vi "Lab6_template_v1.0.vi"() -> ()   [LabVIEW 2018]
doc: "Main VI for the controls"
uses:
  components/PMCL Dynamic Signal Analyzer/Controls/DSA excitation specs.ctl
  components/PMCL Dynamic Signal Analyzer/Controls/DSA cycle specs.ctl
  Typedefs/StateDef_Enum.ctl
  <vilib>/Utility/error.llb/DialogType.ctl
  components/Motor Read Angle/Task cluster.ctl
  <vilib>/Platform/TimedLoop/XDataNode/timing_clust.ctl
  <vilib>/Platform/TimedLoop/XDataNode/nitl_modes.ctl
  <vilib>/Platform/TimedLoop/XDataNode/wakeup.ctl
  <vilib>/DAQmx/write.llb/DAQmx Write (Analog 1D DBL NChan 1Samp).vi
  <vilib>/DAQmx/create/channels.llb/DAQmx Create Channel (AO-Voltage-Basic).vi
  <vilib>/DAQmx/miscellaneous.llb/DAQmx Fill In Error Info.vi
  <vilib>/platform/TimedLoop/XDataNode/XDataNode.xnode
  Components/Timing/Timing.lvlib
  <vilib>/Platform/TimedLoop/XDataNode/XDNodeRunTimeDep.lvlib
  <vilib>/Analysis/NI_AALPro.lvlib
  <vilib>/ptbypt/NI_PtbyPt.lvlib
  Components/Controller/Controller.lvlib
  components/Motor Read Angle/Motor_ReadAng.lvlib
panel:
  in  "System Stop Button":bool
  in  "Pause chart?":bool
  in  "Controller Params":enum32{"Page 1"}(tab)
  in  "Kp":dbl=1.0 min=0.0
  in  "Controller On?":bool
  out "Found index?":bool
  out "Status":string="Stopped."
  in  "Ref. Gen.":T1(tab)=enum."Manual"
  in  "Ref. cmd.":dbl(slide) caption="Ref. cmd. [deg.]" step=1.0 scale=-90.0..90.0 scale format="%#.1f"
  in  "Signal Cluster":T2={"phase"=0.0, "amplitude"=1.0, "frequency"=1.0, "offset"=1.0, "Signal"=enum."Square"} {"offset" format="%0.2f"; "frequency" format="%0.2f"; "amplitude" format="%0.2f"; "phase" format="%0.2f"}
  in  "Frequency\nResponse":enum16{"Plant", "RR", "CL"}(ring)
  out "DSA \nRunning?":bool
  in  "Stop \nDSA":bool
  in  "Start \nDSA":bool
  in  "DSA excitation specs":T3={"Initial Freq. [Hz]"=10.0, "Final Freq. [Hz]"=999.0, "# pts. in interval"=50, "Samping Time [s]"=0.000333, "Amplitude [V]"=1.0, "Offset [V]"=0.0, "Freq Units (F: rad/s, T: Hz)"=TRUE}
  in  "Cycle Specs":T4={"Cycles To \nSettle (M)"=5, "Cycles To \nCalculate (N)"=10}
  in  "Loop Timing":enum32{"Comm.", "Ctrl.", "Ref. gen", "UI"}(tab)
  out "# Finished\nLate counter":dbl
  in  "Comm.\nLoop Rate (Hz)":dbl=10000.0 format="%#_4p"
  in  "Ctrl.\nLoop Rate (Hz)":dbl=5000.0 format="%#_4p"
  out "# Finished\nLate counter":dbl
  out "# Finished\nLate counter":dbl
  in  "Ref. Gen.\nLoop Rate (Hz)":dbl=3000.0 format="%#_4p"
  in  "UI Loop rate (Hz)":dbl=100.0 format="%#_6p"
  in  "Display Waveforms":enum32{"Controller Signals", "DSA "}(tab)
  out "Control Effort":T5(graph)={"Double"=0.0, "Double"=-0.0, "Double"=0.0}
  out "Waveform Chart":T6(graph)
  out "Phase Bode Plot":cluster{dbl[], dbl[]}(graph)
  out "Magnitude Bode Plot":cluster{dbl[], dbl[]}(graph)
  out "DSA Signals":cluster{"Double":dbl, "Double":dbl}(graph)
  # "Connect the Reference Signal \nto C/AI 1 of the myRIO."
  # "Pinout Config.:\nPort C/AI0 : Plant output being read           by the controller.\nPort C/AI1 : Reference signal for the control loop.\nPort C/AO0 : Control effort signal to the plant."
  # "Implement Trajectory Generation \nUI elements here"
  # "Commutation Loop Timing"
  # "Control Loop Timing"
  # "Ref.  Gen. Loop Timing"
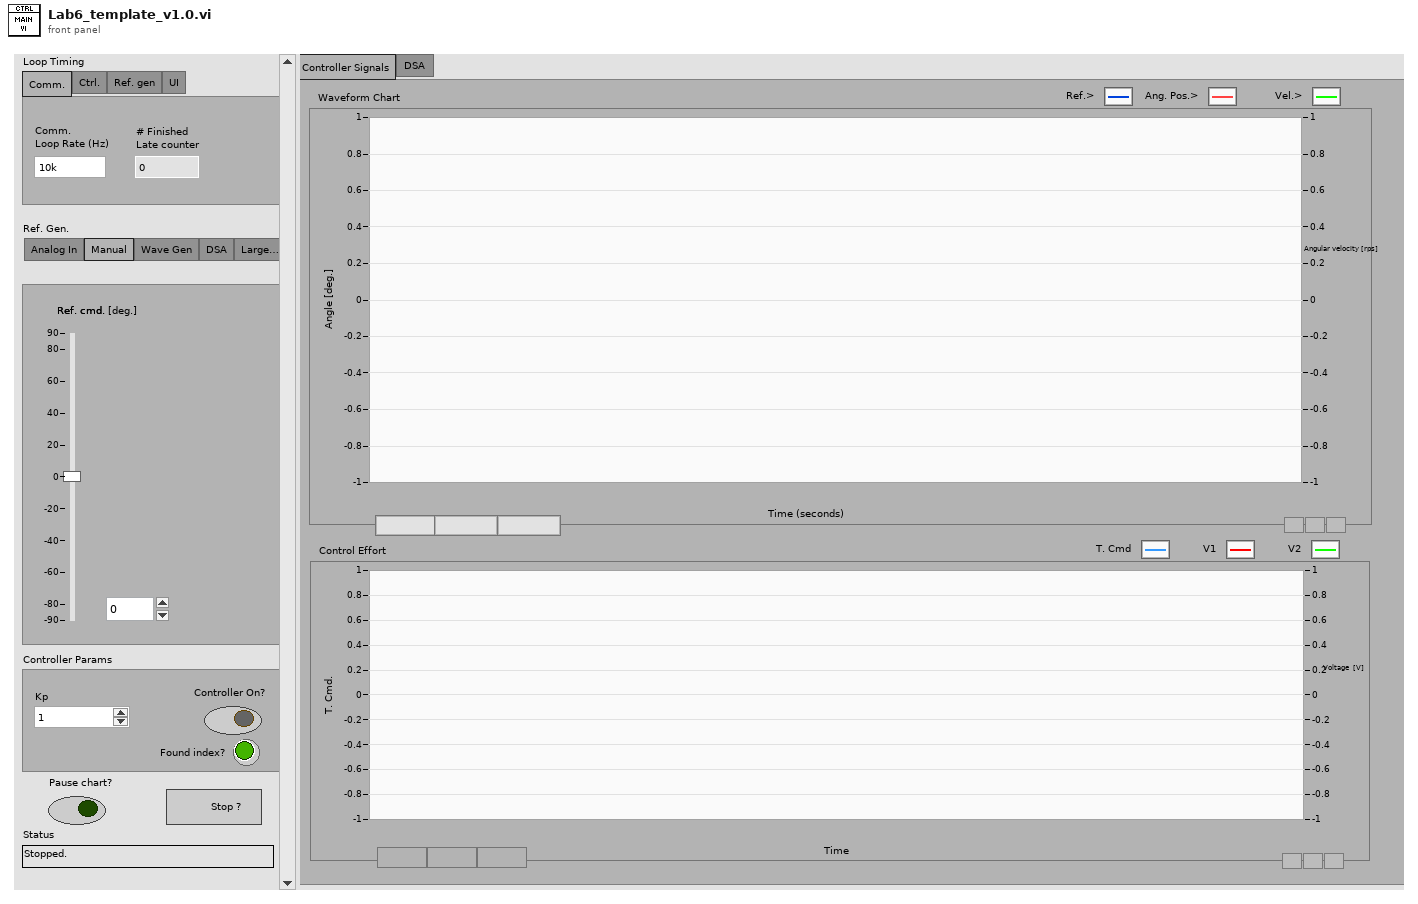
[diagram p1: front panel]
types:
  T1 = enum32{"Analog In", "Manual", "Wave Gen", "DSA", "Large Step"}
  T2 = cluster{"phase":dbl, "amplitude":dbl, "frequency":dbl, "offset":dbl, "Signal":enum16{"Sine", "Square", "Sawtooth"}}
  T3 = typedef "DSA excitation specs.ctl" = cluster{"Initial Freq. [Hz]":dbl, "Final Freq. [Hz]":dbl, "# pts. in interval":i16, "Samping Time [s]":dbl, "Amplitude [V]":dbl, "Offset [V]":dbl, "Freq Units (F: rad/s, T: Hz)":bool}
  T4 = typedef "DSA cycle specs.ctl" = cluster{"Cycles To \nSettle (M)":i16, "Cycles To \nCalculate (N)":i16}
  T5 = cluster{"Double":dbl, "Double":dbl, "Double":dbl}
  T6 = cluster{"Double":dbl, "Numeric":dbl, "Numeric":dbl}
  T7 = typedef "Motor_ReadAng.lvlib/Task cluster.ctl" = cluster{"DAQmx Task Enc1":refnum<k21>, "DAQmx Task EncRef1":refnum<k21>, "DAQmx Task Enc2":refnum<k21>, "DAQmx Task EncRef2":refnum<k21>}
  T8 = typedef "DialogType.ctl" = u16
  T9 = typedef "StateDef_Enum.ctl" = enum16{"Initialize", "Wait", "Shutdown"}
  T10 = typedef "XDNodeRunTimeDep.lvlib/timing_clust.ctl" = cluster{"Expected End [f-1]":u64, "Actual End [f-1]":u64, "Finished Late? [f-1]":bool, "Expected End [i-1]":u64, "Actual End [i-1]":u64, "Finished Late? [i-1]":bool, "Expected Start [i]":u64, "Actual Start [i]":u64, "Expected Start [f]":u64, "Actual Start [f]":u64, "Source Name":string, "Structure Name":string, "Period":i64, "Deadline":i64, "Offset":i64, "Start":i64, "Priority":i32, "Timeout":i32, "Mode":T11, "Wakeup Reason":T12, "Error":errorcluster, "Source Type":string, "Secondary Source Type":string, "Global End Time":u64, "Global Start Time":u64, "Frame Duration":u64, "Iteration Duration":u64, "Assigned CPU":i32, "I/O Scan Engine Mode":u32}
  T11 = typedef "XDNodeRunTimeDep.lvlib/nitl_modes.ctl" = enum32{"No Change", "Process missed periods, maintain original phase", "Discard missed periods, maintain original phase", "Process missed periods, ignore original phase", "Discard missed periods, ignore original phase"}
  T12 = typedef "XDNodeRunTimeDep.lvlib/wakeup.ctl" = enum32{"Normal", "Aborted", "Asynchronous wakeup", "Timing source error", "Timed loop error", "Timeout"}
  T13 = cluster{"Analog In CH1":dbl, "Analog In CH0":dbl}
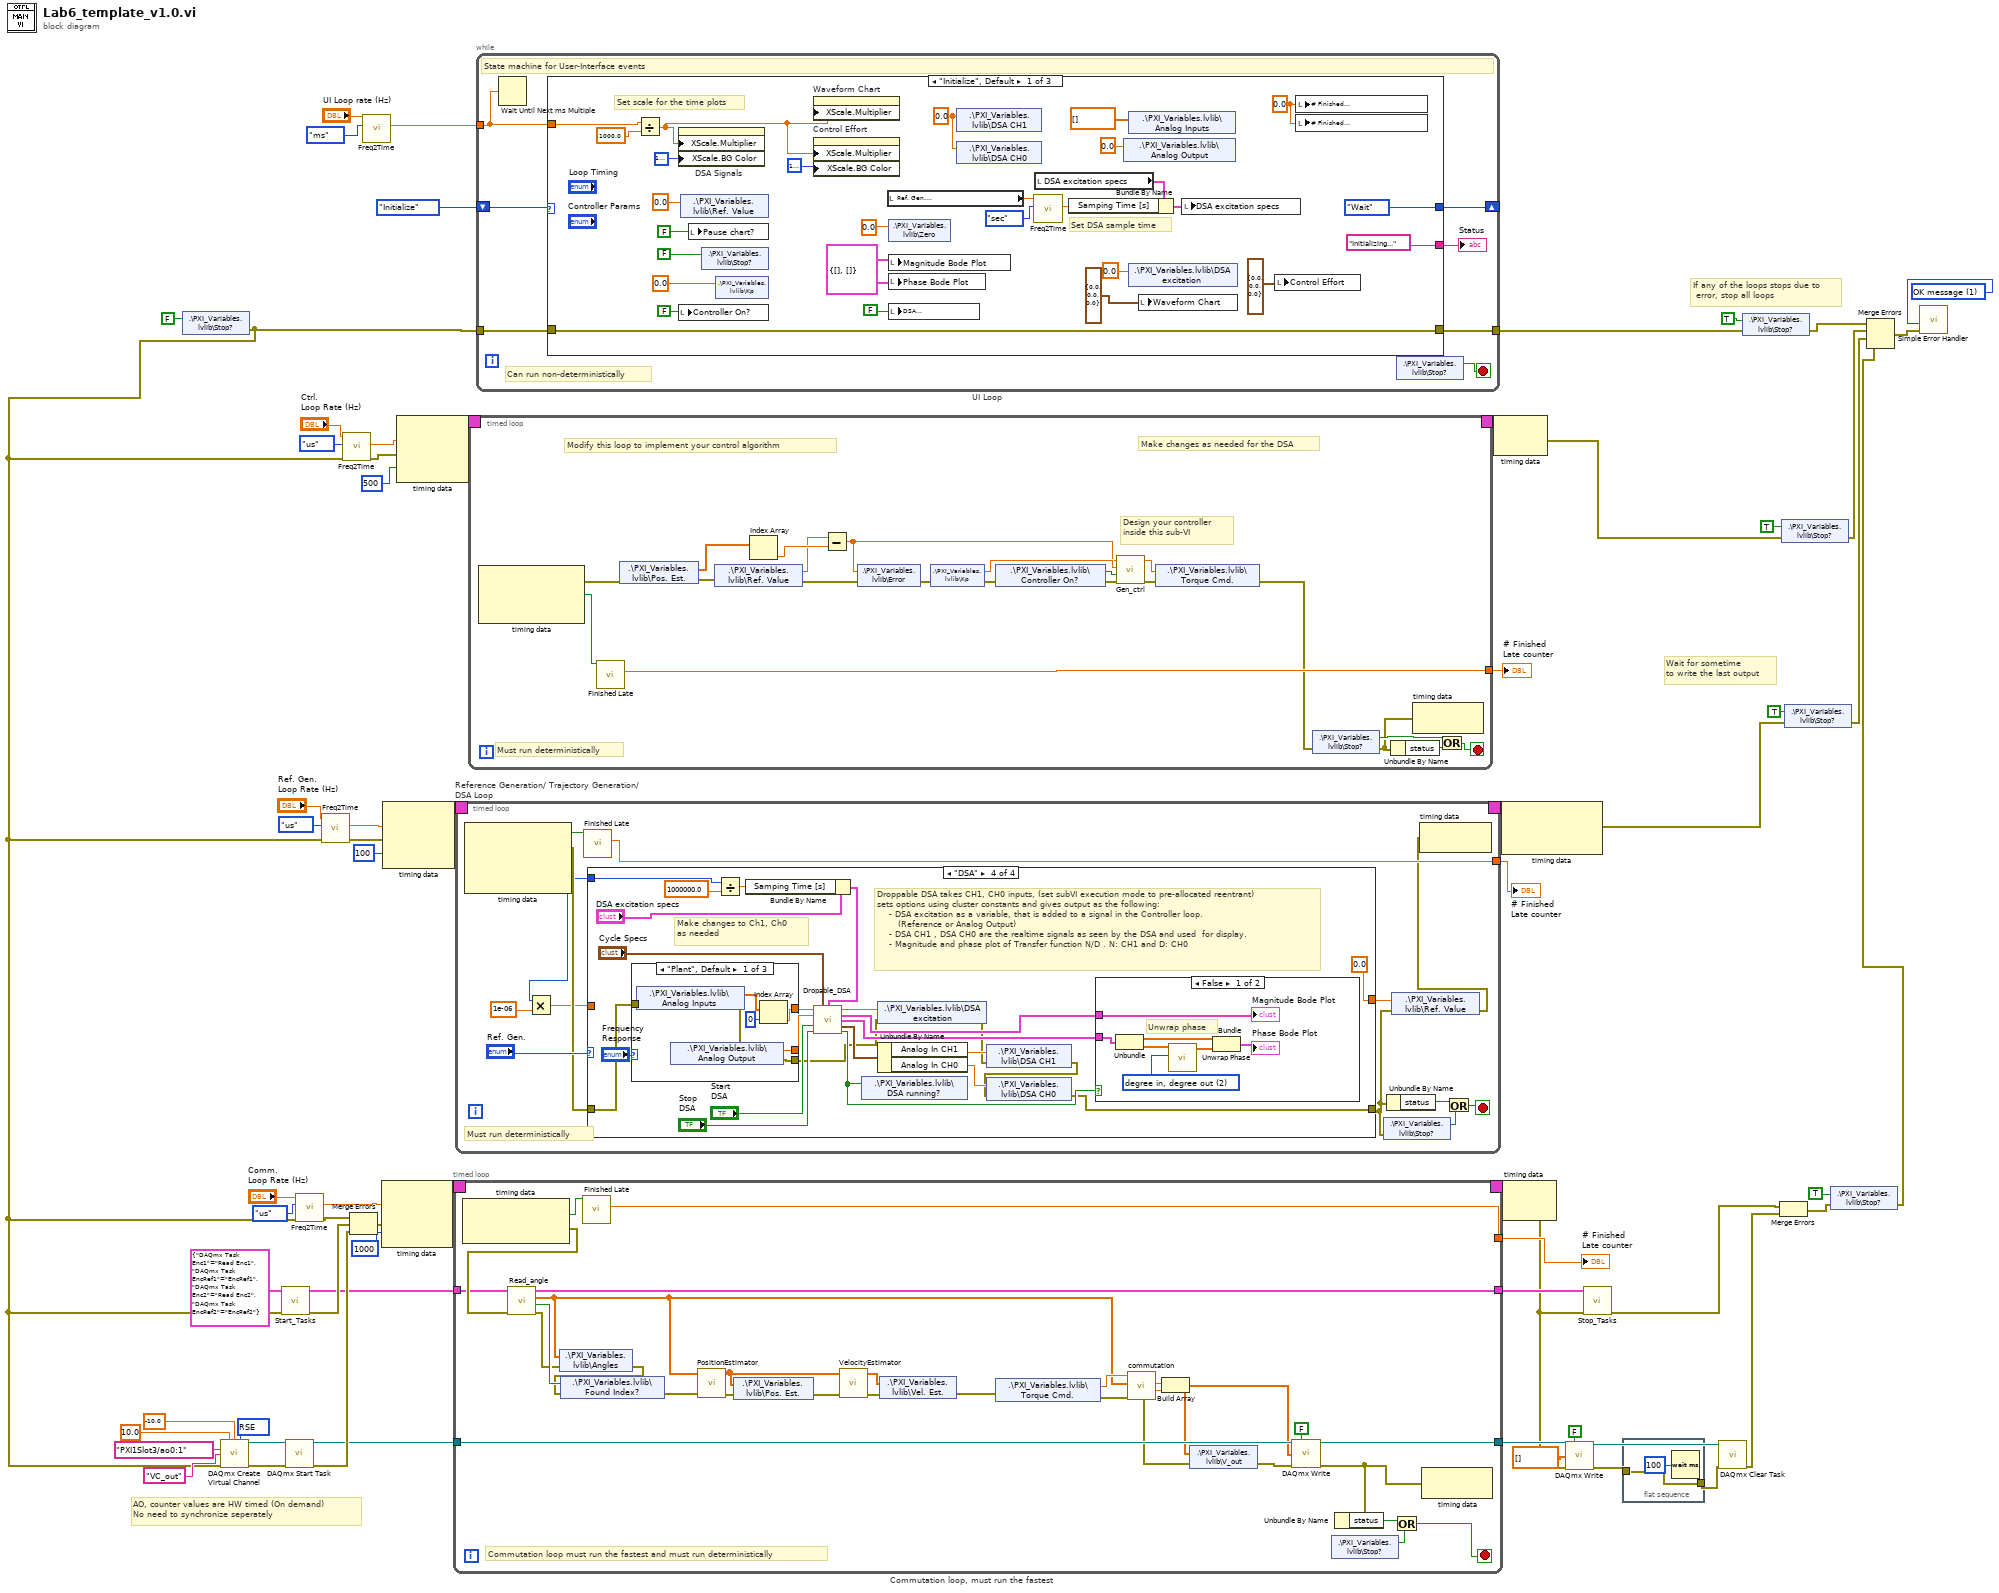
[diagram p0: block diagram]
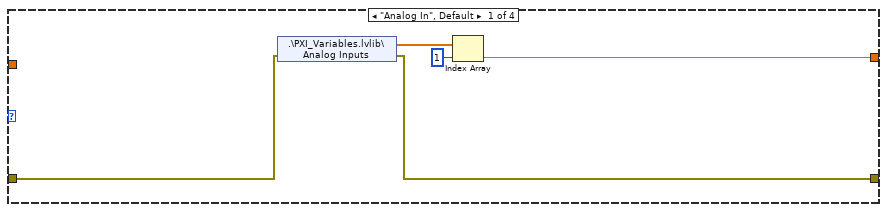
[diagram p2: hidden frame]
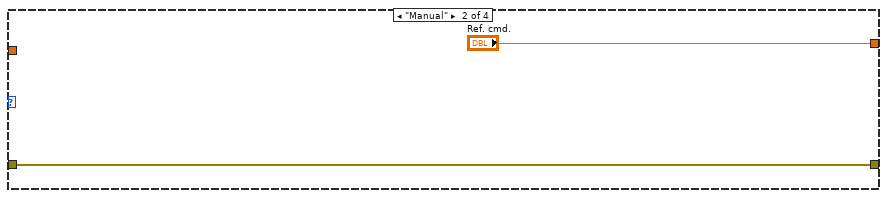
[diagram p3: hidden frame]
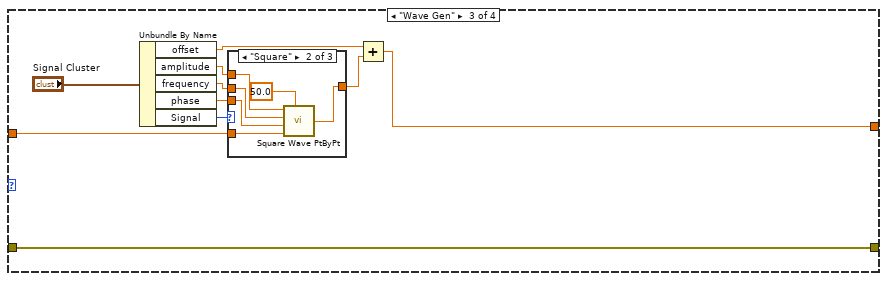
[diagram p4: hidden frame]
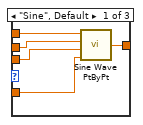
[diagram p5: hidden frame]
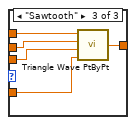
[diagram p6: hidden frame]
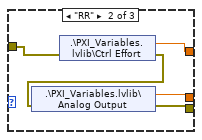
[diagram p7: hidden frame]
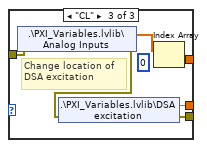
[diagram p8: hidden frame]
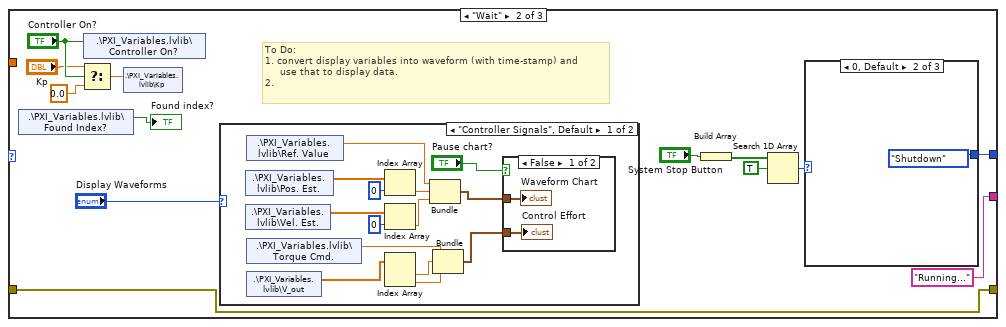
[diagram p10: hidden frame]
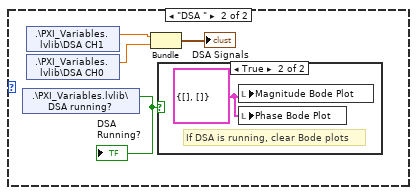
[diagram p12: hidden frame]
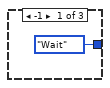
[diagram p14: hidden frame]
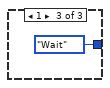
[diagram p15: hidden frame]
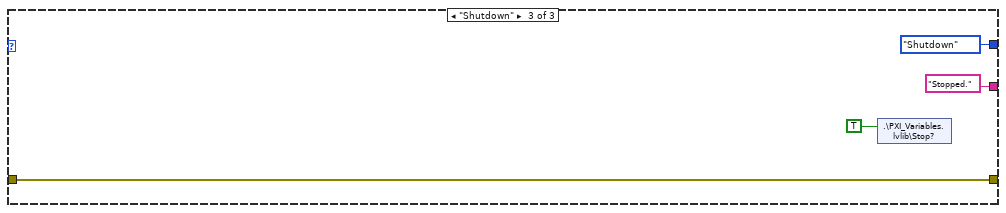
[diagram p16: hidden frame]
diagram:
  w35 = 10083 items=["Default"=-1, "RSE"=10083, "Differential"=10106, "Pseudodifferential"=12529] ("output terminal configuration")
  w48 = T8 1 items=["no dialog", "OK message", "continue or stop message", "OK message + warnings", "continue/stop + warnings"] ("type of dialog (OK msg:1)")
  # "AO, counter values are HW timed (On demand)\nNo need to synchronize seperately"
  # "Wait for sometime \nto write the last output"
  # "If any of the loops stops due to\n error, stop all loops"
  n1 = shared-variable ".\\PXI_Variables.lvlib\\Stop?"(FALSE ("Stop?")) -> (error out=w22:errorcluster)  [unwired: 1 in]
  n2 = call-poly <vilib>:"DAQmx Create Virtual Channel.vi"("maximum value"=10.0, "minimum value"=-10.0, "output terminal configuration"=w35, "physical channels"=tag "PXI1Slot3/ao0:1", "name to assign"="VC_out", "error in"=w22) -> ("task out"=w33:refnum<k21>, "error out"=w32:errorcluster)  [unwired: 8 in]
  n3 = call "Start_Tasks.vi"("error in (no error)"=w22, "Task cluster In"=T7 {"DAQmx Task Enc1"="Read Enc1", "DAQmx Task EncRef1"="EncRef1", "DAQmx Task Enc2"="Read Enc2", "DAQmx Task EncRef2"="EncRef2"}) -> ("error out"=w25:errorcluster, "Task cluster Out"=w21:T7)  [unwired: 8 in]
  n4 = call <vilib>:"DAQmx Start Task.vi"("task/channels in"=w33, "error in"=w32) -> ("task out"=w17:refnum<k21>, "error out"=w24:errorcluster)  [unwired: 12 in]
  n5 = call "Freq2Time.vi"("error in (no error)"=w22, "Int. Time Unit"=enum16{"sec", "us", "ms"}."us", "Sample rate (Hz)"="Comm.\nLoop Rate (Hz)") -> ("error out"=w26:errorcluster, "Int.  time [unit]"=w41:dbl)  [unwired: 6 in, 1 out]
  n6 = call "Freq2Time.vi"("error in (no error)"=w22, "Int. Time Unit"=enum16{"sec", "us", "ms"}."us", "Sample rate (Hz)"="Ref. Gen.\nLoop Rate (Hz)") -> ("error out"=w42:errorcluster, "Int.  time [unit]"=w47:dbl)  [unwired: 6 in, 1 out]
  n7 = call "Freq2Time.vi"("error in (no error)"=w22, "Int. Time Unit"=enum16{"sec", "us", "ms"}."us", "Sample rate (Hz)"="Ctrl.\nLoop Rate (Hz)") -> ("error out"=w31:errorcluster, "Int.  time [unit]"=w1:dbl)  [unwired: 6 in, 1 out]
  n8 = Merge Errors(w26, w25, w24) -> (w27:errorcluster)
  n9 = call "Freq2Time.vi"("Int. Time Unit"=enum16{"sec", "us", "ms"}."ms", "Sample rate (Hz)"="UI Loop rate (Hz)") -> ("Int.  time [unit]"=w58:dbl)  [unwired: 7 in, 2 out]
  n10 = node-c288(w41, w27, 1000 ("Priority")) -> (w44:T10)
  n11 = node-c288(w47, w42, 100 ("Priority")) -> (w65:T10)
  n12 = node-c288(w1, w31, 500 ("Priority")) -> (w53:T10)
  n13 = timed-loop "Commutation loop, must run the fastest" {
    timing: w44 -> [_]
    timing-out: [_] -> w43
    tunnel: [w96] -> w39
    tunnel: w21 -> [w94]
    tunnel: [w86] -> w16
    tunnel: w17 -> [w87]
    tunnel: [w93] -> w10
    stop <- w80 stop-if-true
    # "Commutation loop must run the fastest and must run deterministically"
    n14 = node-c288() -> (w97:bool, w95:errorcluster)  [unwired: 1 in]
    n15 = call "Read_angle.vi"("error in (no error)"=w95, "Task cluster In"=w94) -> ("error out"=w91:errorcluster, "Found index?"=w92:bool, "appended array"=w78:dbl[], "Task cluster Out"=w93:T7)  [unwired: 6 in]
    n16 = shared-variable ".\\PXI_Variables.lvlib\\Angles"(w78, error in=w91) -> (error out=w90:errorcluster)
    n17 = shared-variable ".\\PXI_Variables.lvlib\\Found Index?"(w92, error in=w90) -> (error out=w77:errorcluster)
    n18 = call "Finished Late.vi"("Finished \nLate?"=w97) -> ("# Finished\nLate counter"=w96:dbl)  [unwired: 8 in, 2 out]
    n19 = call "PositionEstimator.vi"("error in (no error)"=w77, "Angles In"=w78) -> ("error out"=w76:errorcluster, "Positions Out"=w69:dbl[])  [unwired: 8 in]
    n20 = shared-variable ".\\PXI_Variables.lvlib\\Pos. Est."(w69, error in=w76) -> (error out=w72:errorcluster)
    n21 = call "VelocityEstimator.vi"("error in (no error)"=w72, "Position In"=w69) -> ("error out"=w71:errorcluster, "Vel. Out"=w68:dbl[])  [unwired: 8 in]
    n22 = shared-variable ".\\PXI_Variables.lvlib\\Vel. Est."(w68, error in=w71) -> (error out=w70:errorcluster)
    n23 = shared-variable ".\\PXI_Variables.lvlib\\Torque Cmd."(error in=w70) -> (w89:dbl, error out=w88:errorcluster)
    n24 = call "commutation.vi"("error in (no error)"=w88, "Theta [deg] Array In"=w78, "Torque Cmd - Td [Ncm]"=w89) -> ("error out"=w74:errorcluster, "Voltage 2 [V]"=w84:dbl, "Voltage 1 [V]"=w85:dbl)  [unwired: 6 in]
    n25 = Build Array(w85, w84) -> (w75:dbl[])
    n26 = shared-variable ".\\PXI_Variables.lvlib\\V_out"(w75, error in=w74) -> (error out=w73:errorcluster)
    n27 = call-poly <vilib>:"DAQmx Write.vi"("task/channels in"=w87, "auto start"=FALSE, "data"=w75, "error in"=w73) -> ("task out"=w86:refnum<k21>, "error out"=w79:errorcluster)  [unwired: 9 in, 1 out]
    n28 = shared-variable ".\\PXI_Variables.lvlib\\Stop?"() -> (w82:bool)  [unwired: 1 in, 1 out]
    n29 = Unbundle By Name(w79) -> ("status"=w83:bool)
    n30 = Or(x=w83, y=w82) -> (x .or. y?=w80:bool)
    n31 = node-c288(w79) -> ()  [unwired: 1 out]
  }
  "# Finished\nLate counter" <- w39
  n32 = timed-loop "Reference Generation/ Trajectory Generation/ DSA Loop" {
    timing: w65 -> [_]
    timing-out: [_] -> w64
    tunnel: [w116] -> w63
    stop <- w110 stop-if-true
    # "Must run deterministically"
    n33 = node-c288() -> (w117:bool, w113:errorcluster, w107:i64, w106:i64)  [unwired: 1 in]
    n34 = Multiply(x=w107, y=1e-06) -> (x*y=w109:dbl)
    n35 = call "Finished Late.vi"("Finished \nLate?"=w117) -> ("# Finished\nLate counter"=w116:dbl)  [unwired: 8 in, 2 out]
    n36 = case shown="\"DSA\"" "Ref. Gen." {
      tunnel: [w122 "Ref. cmd." w127 0.0 ("Ref. cmd.")] -> w114
      tunnel: w113 -> [w120 w123 w126 w152]
      tunnel: [w119 w123 w126 w158] -> w104
      tunnel: w109 -> [_ _ w125 _]
      tunnel: w106 -> [_ _ _ w165]
      frame "Analog In", Default {
        n37 = shared-variable ".\\PXI_Variables.lvlib\\Analog Inputs"(error in=w120) -> (w121:dbl[], error out=w119:errorcluster)
        n38 = Index Array(array=w121, index=1) -> (element=w122:dbl)
      }
      frame "Manual" {
      }
      frame "Wave Gen" {
        n39 = Unbundle By Name("Signal Cluster") -> ("offset"=w128:dbl, "amplitude"=w131:dbl, "frequency"=w130:dbl, "phase"=w129:dbl, "Signal"=w132:enum16{"Sine", "Square", "Sawtooth"})
        n40 = case shown="\"Square\"" w132 {
          tunnel: [w139 w144 w150] -> w134
          tunnel: w131 -> [w138 w143 w149]
          tunnel: w130 -> [w137 w142 w148]
          tunnel: w129 -> [w136 w141 w147]
          tunnel: w125 -> [w135 w140 w146]
          frame "Sine", Default {
            n41 = call <vilib>:"Sine Wave PtByPt.vi"("time"=w135, "phase"=w136, "frequency"=w137, "amplitude"=w138) -> ("sine wave"=w139:dbl)
          }
          frame "Square" {
            n42 = call <vilib>:"Square Wave PtByPt.vi"("amplitude"=w143, "frequency"=w142, "phase"=w141, "time"=w140, "duty cycle (%)"=50.0) -> ("square wave"=w144:dbl)
          }
          frame "Sawtooth" {
            n43 = call <vilib>:"Triangle Wave PtByPt.vi"("time"=w146, "phase"=w147, "frequency"=w148, "amplitude"=w149) -> ("triangle wave"=w150:dbl)
          }
        }
        n44 = Add(x=w128, y=w134) -> (x+y=w127:dbl)
      }
      frame "DSA" {
        # "Make changes to Ch1, Ch0 \nas needed"
        # "Droppable DSA takes CH1, CH0 inputs, (set subVI execution mode to pre-allocated reentrant) \nsets options using cluster constants and gives output as the following:\n    - DSA excitation as a variable, that is added to a signal in the Controller loop. \n       (Reference or Analog Output)\n    - DSA CH1 , DSA CH0 are the realtime signals as seen by the DSA and used  for display.\n    - Magnitude and phase plot of Transfer function N/D . N: CH1 and D: CH0"
        n45 = case shown="\"Plant\", Default" "Frequency\nResponse" {
          tunnel: [w181 w186 w191] -> w156
          tunnel: [w180 w185 w192] -> w153
          tunnel: w152 -> [w177 w183 w190]
          tunnel: [w175 w182 w188] -> w151
          frame "Plant", Default {
            n46 = shared-variable ".\\PXI_Variables.lvlib\\Analog Inputs"(error in=w177) -> (w178:dbl[], error out=w176:errorcluster)
            n47 = shared-variable ".\\PXI_Variables.lvlib\\Analog Output"(error in=w176) -> (w181:dbl, error out=w180:errorcluster)
            n48 = Index Array(array=w178, index=0) -> (element=w175:dbl)
          }
          frame "RR" {
            n49 = shared-variable ".\\PXI_Variables.lvlib\\Ctrl Effort"(error in=w183) -> (w182:dbl, error out=w184:errorcluster)
            n50 = shared-variable ".\\PXI_Variables.lvlib\\Analog Output"(error in=w184) -> (w186:dbl, error out=w185:errorcluster)
          }
          frame "CL" {
            (unwired) 0 ("index")
            # "Change location of\nDSA excitation"
            n51 = shared-variable ".\\PXI_Variables.lvlib\\Analog Inputs"(error in=w190) -> (w189:dbl[], error out=w187:errorcluster)
            n52 = shared-variable ".\\PXI_Variables.lvlib\\DSA excitation"(error in=w187) -> (w191:dbl, error out=w192:errorcluster)
            n53 = Index Array(array=w189) -> (element=w188:dbl)  [unwired: 1 in]
          }
        }
        n54 = Divide(x=w165, y=1000000.0) -> (x/y=w163:dbl)
        n55 = Bundle By Name(cluster="DSA excitation specs", "Samping Time [s]"=w163) -> (w162:T3)
        n56 = call "Dropable_DSA.vi"("Analog In CH1"=w151, "Cycle Specs"="Cycle Specs", "Excitation Specs"=w162, "Analog In CH0"=w156, "START"="Start \nDSA", "STOP"="Stop \nDSA") -> ("Analog Out"=w173:dbl, "Bode Magnitude"=w167:cluster{dbl[], dbl[]}, "Bode Phase"=w166:cluster{dbl[], dbl[]}, "Live signals"=w170:T13, "Running"=w161:bool)  [unwired: 4 in, 1 out]
        n57 = shared-variable ".\\PXI_Variables.lvlib\\DSA running?"(w161) -> ()  [unwired: 1 in, 1 out]
        n58 = shared-variable ".\\PXI_Variables.lvlib\\DSA excitation"(w173, error in=w153) -> (error out=w160:errorcluster)
        n59 = Unbundle By Name(w170) -> ("Analog In CH1"=w169:dbl, "Analog In CH0"=w168:dbl)
        n60 = shared-variable ".\\PXI_Variables.lvlib\\DSA CH1"(w169, error in=w160) -> (error out=w159:errorcluster)
        n61 = shared-variable ".\\PXI_Variables.lvlib\\DSA CH0"(w168, error in=w159) -> (error out=w158:errorcluster)
        n62 = case shown="False" w161 {
          tunnel: w167 -> [w193 _]
          tunnel: w166 -> [w195 _]
          frame False {
            w197 = 2 items=["radian in, radian out", "radian in, degree out", "degree in, degree out", "degree in, radian out"] ("phase unit")
            # "Unwrap phase"
            n63 = Unbundle(w195) -> (w199:dbl[], w196:dbl[])
            n64 = call <vilib>:"Unwrap Phase.vi"("phase unit"=w197, "Phase"=w196) -> ("Unwrapped Phase"=w198:dbl[])  [unwired: 8 in, 1 out]
            n65 = Bundle(w199, "Unwrapped Phase"=w198) -> (→"Phase Bode Plot":cluster{dbl[], "Unwrapped Phase":dbl[]})  [unwired: 1 in]
            "Magnitude Bode Plot" <- w193
          }
          frame True {
          }
        }
      }
    }
    n66 = shared-variable ".\\PXI_Variables.lvlib\\Stop?"(error in=w104) -> (w111:bool)  [unwired: 1 out]
    n67 = Unbundle By Name(w104) -> ("status"=w112:bool)
    n68 = shared-variable ".\\PXI_Variables.lvlib\\Ref. Value"(w114, error in=w104) -> (error out=w105:errorcluster)
    n69 = node-c288(w105) -> ()  [unwired: 1 out]
    n70 = Or(x=w112, y=w111) -> (x .or. y?=w110:bool)
  }
  "# Finished\nLate counter" <- w63
  n71 = timed-loop {
    timing: w53 -> [_]
    timing-out: [_] -> w52
    tunnel: [w227] -> w49
    stop <- w223 stop-if-true
    # "Make changes as needed for the DSA"
    # "Modify this loop to implement your control algorithm"
    # "Must run deterministically"
    # "Design your controller \ninside this sub-VI"
    n72 = node-c288() -> (w210:errorcluster, w228:bool)  [unwired: 1 in, 1 out]
    n73 = call "Finished Late.vi"("Finished \nLate?"=w228) -> ("# Finished\nLate counter"=w227:dbl)  [unwired: 8 in, 2 out]
    n74 = shared-variable ".\\PXI_Variables.lvlib\\Pos. Est."(error in=w210) -> (w209:dbl[], error out=w208:errorcluster)
    n75 = shared-variable ".\\PXI_Variables.lvlib\\Ref. Value"(error in=w208) -> (w218:dbl, error out=w212:errorcluster)
    n76 = Index Array(array=w209) -> (element=w219:dbl)  [unwired: 1 in]
    n77 = Subtract(x=w218, y=w219) -> (x-y=w213:dbl)
    n78 = shared-variable ".\\PXI_Variables.lvlib\\Error"(w213, error in=w212) -> (error out=w211:errorcluster)
    n79 = shared-variable ".\\PXI_Variables.lvlib\\Kp"(error in=w211) -> (w217:dbl, error out=w215:errorcluster)
    n80 = shared-variable ".\\PXI_Variables.lvlib\\Controller On?"(error in=w215) -> (w216:bool, error out=w214:errorcluster)
    n81 = call "Gen_ctrl.vi"("error in (no error)"=w214, "Controller On?"=w216, "Kp"=w217, "Error In"=w213) -> ("error out"=w222:errorcluster, "Ctrl Effort Out"=w220:dbl)  [unwired: 6 in]
    n82 = shared-variable ".\\PXI_Variables.lvlib\\Torque Cmd."(w220, error in=w222) -> (error out=w221:errorcluster)
    n83 = shared-variable ".\\PXI_Variables.lvlib\\Stop?"(error in=w221) -> (w226:bool, error out=w225:errorcluster)
    n84 = Unbundle By Name(w225) -> ("status"=w224:bool)
    n85 = node-c288(w225) -> ()  [unwired: 1 out]
    n86 = Or(x=w226, y=w224) -> (x .or. y?=w223:bool)
  }
  "# Finished\nLate counter" <- w49
  n87 = while "UI Loop" {
    shift-right: [w240] -> _
    shift-left: StateDef_Enum."Initialize" ("State defining Enum") -> [w241]
    tunnel: w22 -> [w239]
    tunnel: [w238] -> w57
    tunnel: w58 -> [w235]
    stop <- w236 stop-if-true
    # "Can run non-deterministically"
    # "State machine for User-Interface events"
    n88 = Wait Until Next ms Multiple(millisecond multiple=w235) -> ()  [unwired: 1 out]
    n89 = case shown="\"Initialize\", Default" w241 {
      tunnel: [StateDef_Enum."Wait" ("State defining Enum") w279 StateDef_Enum."Shutdown" ("State defining Enum")] -> w240
      tunnel: w239 -> [w266 w277 w310]
      tunnel: [w266 w277 w310] -> w238
      tunnel: ["Initializing..." ("Status") "Running..." ("Status") "Stopped." ("Status")] -> w237
      tunnel: w235 -> [w264 _ _]
      frame "Initialize", Default {
        w244 = 0.0 ("# Finished\nLate counter")
        w245 = 0.0 ("DSA CH1")
        w259 = cluster{dbl[], dbl[]} {[], []} ("Magnitude Bode Plot")
        # "Set DSA sample time"
        # "Set scale for the time plots"
        n90 = Divide(x=w264, y=1000.0) -> (x/y=w251:dbl)
        n91 = property on="DSA Signals" class="WFChart (strict)"("XScale.Multiplier"=w251, "XScale.BG Color"=u32 16777216) -> ()  [unwired: 2 in, 2 out]
        n92 = local write "Controller On?"(FALSE ("Controller On?")) -> ()
        n93 = shared-variable ".\\PXI_Variables.lvlib\\Ref. Value"(0.0 ("Ref. Value")) -> ()  [unwired: 1 in, 1 out]
        n94 = local write "Pause chart?"(FALSE ("Pause chart?")) -> ()
        n95 = shared-variable ".\\PXI_Variables.lvlib\\Stop?"(FALSE ("Stop?")) -> ()  [unwired: 1 in, 1 out]
        n96 = shared-variable ".\\PXI_Variables.lvlib\\Kp"(0.0 ("Kp")) -> ()  [unwired: 1 in, 1 out]
        n97 = property on="Waveform Chart" class="WFChart (strict)"("XScale.Multiplier"=w251) -> ()  [unwired: 2 in, 2 out]
        n98 = property on="Control Effort" class="WFChart (strict)"("XScale.Multiplier"=w251, "XScale.BG Color"=u32 16777216) -> ()  [unwired: 2 in, 2 out]
        n99 = local read "Ref. Gen.\nLoop Rate (Hz)"() -> (w254:dbl)
        n100 = shared-variable ".\\PXI_Variables.lvlib\\Zero"(0.0 ("Zero")) -> ()  [unwired: 1 in, 1 out]
        n101 = local write "Magnitude Bode Plot"(w259) -> ()
        n102 = local write "Phase Bode Plot"(w259) -> ()
        n103 = local write "DSA \nRunning?"(FALSE ("DSA \nRunning?")) -> ()
        n104 = shared-variable ".\\PXI_Variables.lvlib\\DSA CH1"(w245) -> ()  [unwired: 1 in, 1 out]
        n105 = shared-variable ".\\PXI_Variables.lvlib\\DSA CH0"(w245) -> ()  [unwired: 1 in, 1 out]
        n106 = call "Freq2Time.vi"("Int. Time Unit"=enum16{"sec", "us", "ms"}."sec", "Sample rate (Hz)"=w254) -> ("Int.  time [unit]"=w252:dbl)  [unwired: 7 in, 2 out]
        n107 = local read "DSA excitation specs"() -> (w256:T3)
        n108 = Bundle By Name(cluster=w256, "Samping Time [s]"=w252) -> (w255:T3)
        n109 = shared-variable ".\\PXI_Variables.lvlib\\Analog Output"(0.0 ("Analog Output")) -> ()  [unwired: 1 in, 1 out]
        n110 = shared-variable ".\\PXI_Variables.lvlib\\Analog Inputs"(dbl[] [] ("Analog Inputs")) -> ()  [unwired: 1 in, 1 out]
        n111 = shared-variable ".\\PXI_Variables.lvlib\\DSA excitation"(0.0 ("DSA excitation")) -> ()  [unwired: 1 in, 1 out]
        n112 = local write "Waveform Chart"(T6 {"Double"=0.0, "Numeric"=0.0, "Numeric"=0.0} ("Waveform Chart")) -> ()
        n113 = local write "DSA excitation specs"(w255) -> ()
        n114 = local write "Control Effort"(T5 {"Double"=0.0, "Double"=0.0, "Double"=0.0} ("Control Effort")) -> ()
        n115 = local write "# Finished\nLate counter"(w244) -> ()
        n116 = local write "# Finished\nLate counter"(w244) -> ()
      }
      frame "Wait" {
        # "To Do:\n1. convert display variables into waveform (with time-stamp) and\n     use that to display data.\n2."
        n117 = shared-variable ".\\PXI_Variables.lvlib\\Found Index?"() -> (→"Found index?":bool)  [unwired: 1 in, 1 out]
        n118 = Select(t="Kp", s="Controller On?", f=0.0) -> (s? t:f=w275:dbl)
        n119 = shared-variable ".\\PXI_Variables.lvlib\\Controller On?"("Controller On?") -> ()  [unwired: 1 in, 1 out]
        n120 = shared-variable ".\\PXI_Variables.lvlib\\Kp"(w275) -> ()  [unwired: 1 in, 1 out]
        n121 = case shown="\"Controller Signals\", Default" "Display Waveforms" {
          frame "Controller Signals", Default {
            n122 = shared-variable ".\\PXI_Variables.lvlib\\Pos. Est."() -> (w296:dbl[])  [unwired: 1 in, 1 out]
            n123 = shared-variable ".\\PXI_Variables.lvlib\\Vel. Est."() -> (w285:dbl[])  [unwired: 1 in, 1 out]
            n124 = shared-variable ".\\PXI_Variables.lvlib\\Ref. Value"() -> (w293:dbl)  [unwired: 1 in, 1 out]
            n125 = shared-variable ".\\PXI_Variables.lvlib\\Torque Cmd."() -> (w289:dbl)  [unwired: 1 in, 1 out]
            n126 = shared-variable ".\\PXI_Variables.lvlib\\V_out"() -> (w288:dbl[])  [unwired: 1 in, 1 out]
            n127 = Index Array(array=w296, index=0) -> (element=w295:dbl)
            n128 = Index Array(array=w285, index=0) -> (element=w283:dbl)
            n129 = Index Array(array=w288) -> (element #1=w287:dbl, element #2=w286:dbl)  [unwired: 2 in]
            n130 = Bundle("Double"=w293, "Numeric"=w295, "Numeric"=w283) -> (w291:T6)  [unwired: 1 in]
            n131 = Bundle("Double"=w289, "Numeric"=w287, "Numeric"=w286) -> (w290:T6)  [unwired: 1 in]
            n132 = case shown="False" "Pause chart?" {
              tunnel: w291 -> [w298 _]
              tunnel: w290 -> [w297 _]
              frame False {
                "Waveform Chart" <- w298
                "Control Effort" <- w297
              }
              frame True {
              }
            }
          }
          frame "DSA " {
            n133 = shared-variable ".\\PXI_Variables.lvlib\\DSA running?"() -> (w299:bool)  [unwired: 1 in, 1 out]
            "DSA \nRunning?" <- w299
            n134 = shared-variable ".\\PXI_Variables.lvlib\\DSA CH1"() -> (w301:dbl)  [unwired: 1 in, 1 out]
            n135 = shared-variable ".\\PXI_Variables.lvlib\\DSA CH0"() -> (w300:dbl)  [unwired: 1 in, 1 out]
            n136 = Bundle("Double"=w301, "Double"=w300) -> (→"DSA Signals":cluster{"Double":dbl, "Double":dbl})  [unwired: 1 in]
            n137 = case shown="True" w299 {
              frame False {
              }
              frame True {
                w303 = cluster{dbl[], dbl[]} {[], []} ("Magnitude Bode Plot")
                # "If DSA is running, clear Bode plots"
                n138 = local write "Magnitude Bode Plot"(w303) -> ()
                n139 = local write "Phase Bode Plot"(w303) -> ()
              }
            }
          }
        }
        n140 = Build Array("System Stop Button") -> (w281:bool[])
        n141 = Search 1D Array(1D array=w281, element=TRUE) -> (index of element=w278:i32)  [unwired: 1 in]
        n142 = case shown="0, Default" w278 {
          tunnel: [StateDef_Enum."Wait" ("State defining Enum") StateDef_Enum."Shutdown" ("State defining Enum") StateDef_Enum."Wait" ("State defining Enum")] -> w279
          frame -1 {
          }
          frame 0, Default {
          }
          frame 1 {
          }
        }
      }
      frame "Shutdown" {
        n143 = shared-variable ".\\PXI_Variables.lvlib\\Stop?"(TRUE) -> ()  [unwired: 1 in, 1 out]
      }
    }
    "Status" <- w237
    n144 = shared-variable ".\\PXI_Variables.lvlib\\Stop?"() -> (w236:bool)  [unwired: 1 in, 1 out]
  }
  n145 = node-c288(w52) -> (w13:errorcluster)
  n146 = node-c288(w64) -> (w62:errorcluster)  [unwired: 1 out]
  n147 = node-c288(w43) -> (w9:errorcluster)
  n148 = call-poly <vilib>:"DAQmx Write.vi"("task/channels in"=w16, "auto start"=FALSE, "data"=dbl[] [], "error in"=w9) -> ("task out"=w18:refnum<k21>, "error out"=w19:errorcluster)  [unwired: 9 in, 1 out]
  n149 = call "Stop_Tasks.vi"("error in (no error)"=w9, "Task cluster In"=w10) -> ("error out"=w6:errorcluster)  [unwired: 8 in, 1 out]
  n150 = flat-sequence {
    tunnel: [w312] -> w15
    tunnel: w19 -> [w312]
    frame #0 {
      n151 = Wait (ms)(milliseconds to wait=u32 100) -> ()  [unwired: 1 out]
    }
  }
  n152 = call <vilib>:"DAQmx Clear Task.vi"("task in"=w18, "error in"=w15) -> ("error out"=w7:errorcluster)  [unwired: 13 in]
  n153 = shared-variable ".\\PXI_Variables.lvlib\\Stop?"(TRUE ("Stop?"), error in=w57) -> (error out=w56:errorcluster)
  n154 = Merge Errors(w6, w7) -> (w8:errorcluster)
  n155 = shared-variable ".\\PXI_Variables.lvlib\\Stop?"(TRUE ("Stop?"), error in=w13) -> (error out=w50:errorcluster)
  n156 = shared-variable ".\\PXI_Variables.lvlib\\Stop?"(TRUE ("Stop?"), error in=w62) -> (error out=w51:errorcluster)
  n157 = shared-variable ".\\PXI_Variables.lvlib\\Stop?"(TRUE ("Stop?"), error in=w8) -> (error out=w5:errorcluster)
  n158 = Merge Errors(w56, w50, w51, w5) -> (w66:errorcluster)
  n159 = call <vilib>:"Simple Error Handler.vi"("type of dialog (OK msg:1)"=w48, "error in (no error)"=w66) -> ()  [unwired: 3 in, 5 out]
